vi "Subpanel close request 26_01_18.vi"(7 "Function":T1=enum."Just check subpanel is closed") -> (3 "Subpanel is closed / Proceed":bool)   [LabVIEW 2017]
uses:
  Typedefs/Subpanel close request.ctl
  Global Variables/General Globals.vi
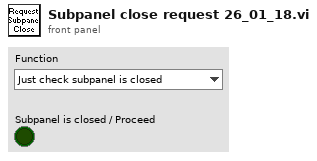
[diagram p1: front panel]
types:
  T1 = typedef "Subpanel close request.ctl" = enum16{"Request subpanel close", "Just check subpanel is closed"}
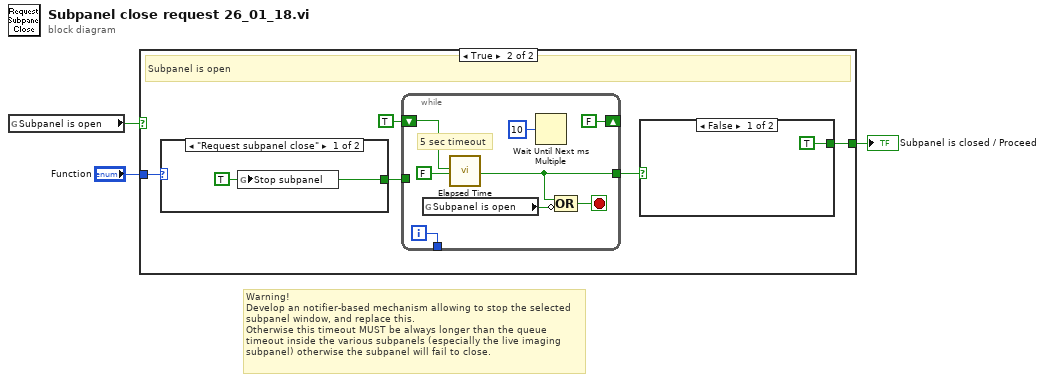
[diagram p0: block diagram]
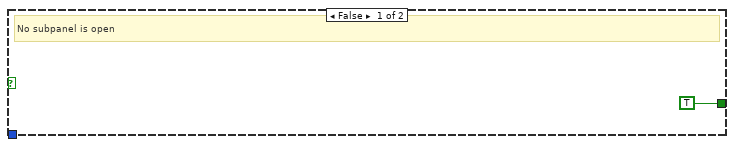
[diagram p2: hidden frame]
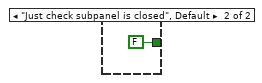
[diagram p3: hidden frame]
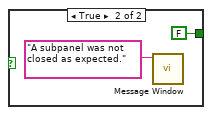
[diagram p4: hidden frame]
diagram:
  # "Warning!\nDevelop an notifier-based mechanism allowing to stop the selected subpanel window, and replace this.\nOtherwise this timeout MUST be always longer than the queue timeout inside the various subpanels (especially the live imaging subpanel) otherwise the subpanel will fail to close."
  n1 = global read "General Globals.vi" "Subpanel is open"() -> (w2:bool)
  n2 = case shown="True" w2 {
    tunnel: [TRUE w6] -> w3
    tunnel: "Function" -> [_ w5]
    frame False {
      # "No subpanel is open"
    }
    frame True {
      # "Subpanel is open"
      n3 = case shown="\"Request subpanel close\"" w5 {
        tunnel: [w10 FALSE ("Stop subpanel")] -> w8
        frame "Request subpanel close" {
          w10 = TRUE ("Stop subpanel")
          n4 = global write "General Globals.vi" "Stop subpanel"(w10) -> ()
        }
        frame "Just check subpanel is closed", Default {
        }
      }
      n5 = while {
        tunnel: [w20] -> w7
        tunnel: [w19] -> _
        shift-right: [FALSE] -> _
        shift-left: TRUE -> [w17]
        tunnel: w8 -> [_]
        i -> [w19]
        stop <- w22 stop-if-true
        # "5 sec timeout"
        n6 = global read "General Globals.vi" "Subpanel is open"() -> (w21:bool)
        n7 = call "Elapsed Time"("Reset"=w17, "Auto Reset"=FALSE) -> ("Time has Elapsed"=w20:bool)  [unwired: 10 in, 7 out]
        n8 = Wait Until Next ms Multiple(millisecond multiple=u32 10) -> ()  [unwired: 1 out]
        n9 = Compound Arithmetic op=OR(w20, invert w21) -> (w22:bool)
      }
      n10 = case shown="False" w7 {
        tunnel: [TRUE FALSE] -> w6
        frame False {
        }
        frame True {
          n11 = call "Message Window.vi"("Message string"="A subpanel was not closed as expected.") -> ()  [unwired: 10 in, 1 out]
        }
      }
    }
  }
  "Subpanel is closed / Proceed" <- w3
